vi "AI RAG Globals.vi"() -> ()   [LabVIEW 2023, in "LabVIEW RAG.lvlib"]
uses:
  LabVIEW RAG.lvlib
panel:
  in  "Tab Control":T1(tab)=enum."Embedding Model"
  in  "ProcessPdfFuncName":string="LoadPdfIntoChromDB"
  in  "RetrContextFuncName":string="RetrieveContextsByUserQuery"
  in  "Python RAG Script":path=path "C:/dev/gaoruhao/ai/src/labview-rag/python/rag.py"
  in  "ProcessMdFuncName":string="ProcessMarkdownFiles"
  in  "Chroma Database Folder":path=path "C:/chroma_db"
  in  "Knowledge Base Name":string="NI-cDAQ"
  in  "Embedding Model URL":string="http://localhost:1234/v1"
  in  "Embedding Model Name":string="mixedbread-ai/mxbai-embed-large-v1"
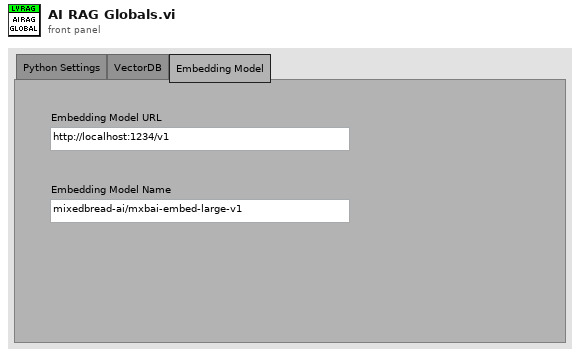
[diagram p1: front panel]
types:
  T1 = enum32{"Python Settings", "VectorDB", "Embedding Model"}
diagram:
